vi "GetExternalInterfaces.vi"(8 "Error In":errorcluster, 11 "reference in":refnum<class "BusBase.lvclass">) -> (0 "Error Out":errorcluster, 2 "ExternalInterfaces":T1[](array[typedef]), 3 "reference out":refnum<class "BusBase.lvclass">)   [LabVIEW 2021, in "BusBase.lvlib" / "BusBase.lvclass"]
uses:
  BusBase.lvclass
  Library_TAF_Support/ClusterArrayConversion/BundledArray.ctl
  e29cbd21-be6e-49f0-8a0b-f762337cc0b1.vi
  <userlib>/_OpenG.lib/lvdata/lvdata.llb/Get Cluster Element Names__ogtk.vi
  Library_TAF_Support/ClusterArrayConversion/ClusterArrayConversion.lvlib
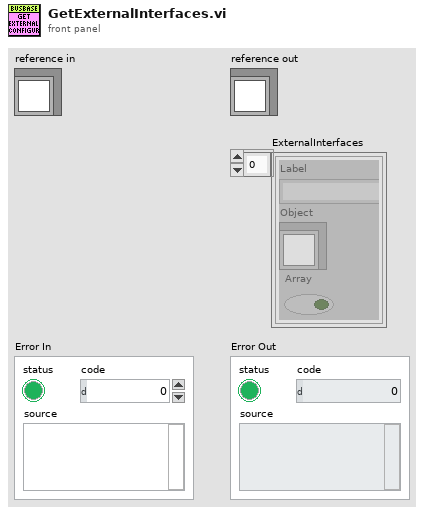
[diagram p1: front panel]
types:
  T1 = typedef "ClusterArrayConversion.lvlib/BundledArray.ctl" = cluster{"Label":string, "Object":refnum<class>, "Array":bool}
  T2 = typedef "BusBase.lvlib/BusBase.lvclass/ObjectAttributes.ctl" = cluster{"Interfaces":cluster{"TargetClasses":refnum<class>[]}, "Locals":cluster{"MainGUIActive":refnum<queue>}, "Persistent":cluster{"Dummy":bool}}
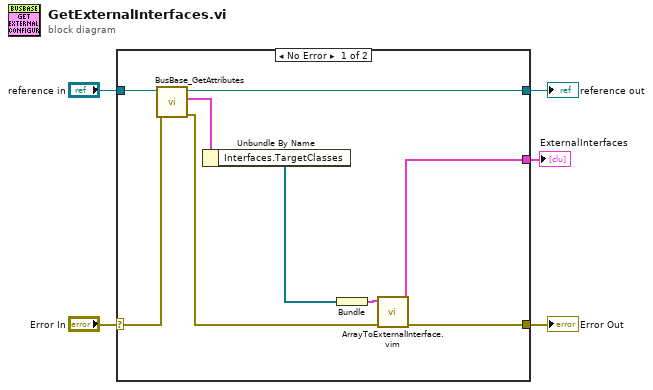
[diagram p0: block diagram]
diagram:
  n1 = case shown="No Error" "Error In" {
    selector: "Error In" -> [w14 w16]
    tunnel: [w9 w16] -> w4
    tunnel: [w11 w15] -> w2
    tunnel: "reference in" -> [w12 w15]
    tunnel: [w10 _] -> w1
    frame No Error {
      n2 = call "BusBase_GetAttributes.vi"("error in (no error)"=w14, "reference in"=w12) -> ("error out"=w8:errorcluster, "Data"=w13:T2, "reference out"=w11:refnum<class "BusBase.lvclass">)  [unwired: 6 in, 1 out]
      n3 = Unbundle By Name(w13) -> ("Interfaces.TargetClasses"=w6:refnum<class>[])
      n4 = Bundle("TargetClasses"=w6) -> (w7:cluster{"TargetClasses":refnum<class>[]})  [unwired: 1 in]
      n5 = call "ArrayToExternalInterface.vim"("error in (no error)"=w8, "Variant"=w7) -> ("error out"=w9:errorcluster, "Array"=w10:T1[])  [unwired: 8 in]
    }
    frame Error {
    }
  }
  "Error Out" <- w4
  "reference out" <- w2
  "ExternalInterfaces" <- w1
